vi "open.local.volume.file.vi"(8 "error in (no error)":errorcluster, 11 "volume json":path) -> (0 "error out":errorcluster, 3 "volume":T1={"id"=0, "name"="", "sortable_name"="", "aliases"=[], "description"="", "site_detail_url"="", "count_of_issues"=0, "start_year"=0, "publisher_id"=0, "issue_ids"=[], "date_last_updated"=timestamp(0 s since 1904-01-01), "volume"=0, "cv_id"="", "volume type"=enum."One Shot"})   [LabVIEW 2024, in "CV_Shared_Library.lvlib"]
uses:
  CV_Shared_Library.lvlib
  CV_RESTful_Library/typedefs/local_volume--cluster.ctl
  volume.type--enum.ctl
  <vilib>/addons/_JKI.lib/Serialization/JSON/JKI JSON Serialization.lvlib
  CV_RESTful_Library/CV_RESTful_Lib.lvlib
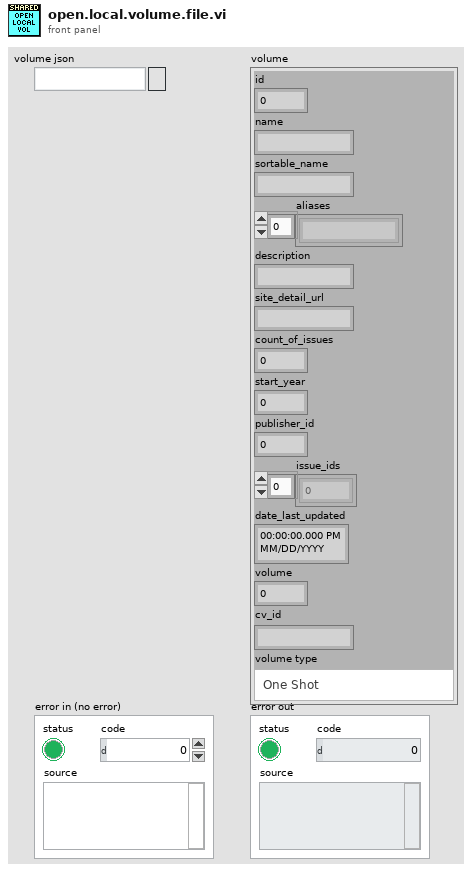
[diagram p1: front panel]
types:
  T1 = typedef "CV_RESTful_Lib.lvlib/local_volume--cluster.ctl" = cluster{"id":i32, "name":string, "sortable_name":string, "aliases":string[], "description":string, "site_detail_url":string, "count_of_issues":i32, "start_year":i32, "publisher_id":i32, "issue_ids":i32[], "date_last_updated":timestamp, "volume":i32, "cv_id":string, "volume type":T2}
  T2 = typedef "CV_Shared_Library.lvlib/volume.type--enum.ctl" = enum16{"Ongoing", "Limited Series", "Annual", "One Shot", "Reprint/Document", "Star Comics", "Epic Comics"}
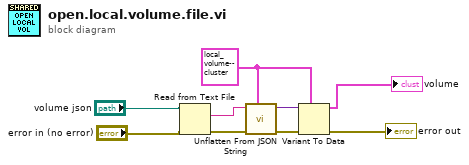
[diagram p0: block diagram]
diagram:
  w6 = T1 {"id"=0, "name"="", "sortable_name"="", "aliases"=[], "description"="", "site_detail_url"="", "count_of_issues"=0, "start_year"=0, "publisher_id"=0, "issue_ids"=[], "date_last_updated"=timestamp(0 s since 1904-01-01), "volume"=0, "cv_id"="", "volume type"=enum."One Shot"} ("volume")
  n1 = Read from Text File(file (use dialog)="volume json", error in="error in (no error)") -> (text=w2:string, error out=w3:errorcluster)  [unwired: 2 in, 2 out]
  n2 = call <vilib>:"Unflatten From JSON String.vi"("Type and Defaults"=w6, "error in"=w3, "JSON String"=w2) -> ("error out"=w4:errorcluster, "Variant"=w5:variant)  [unwired: 7 in]
  n3 = Variant To Data(error in=w4, type=w6, Variant=w5) -> (data=→"volume":T1, error out=→"error out":errorcluster)
